vi "getElementText.vi"(8 "error in (no error)":errorcluster, 11 "xwpfTable in":refnum<class "xwpfTable.lvclass">) -> (0 "error out":errorcluster, 2 "Element.Text":string, 3 "xwpfTable out":refnum<class "xwpfTable.lvclass">)   [LabVIEW 2017, in "Word_Specific.lvlib" / "xwpfTable.lvclass"]
uses:
  xwpfTable.lvclass
  Get Cells.Text
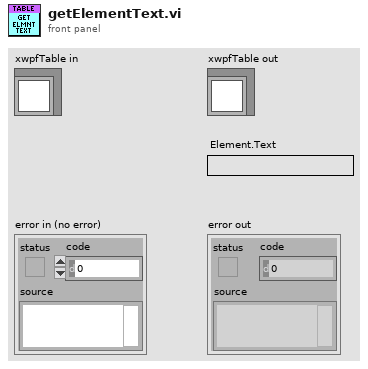
[diagram p1: front panel]
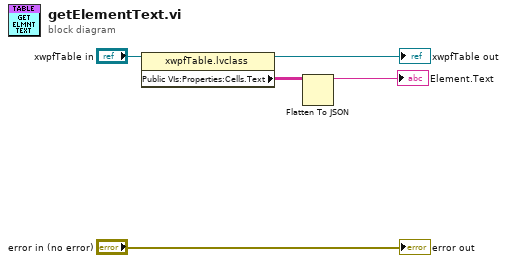
[diagram p0: block diagram]
diagram:
  n1 = property class="xwpfTable.lvclass"(reference="xwpfTable in") -> (reference out=→"xwpfTable out":refnum<class "xwpfTable.lvclass">, "Public VIs:Properties:Cells.Text"=w2:string[][])  [unwired: 1 in, 1 out]
  n2 = Flatten To JSON(anything=w2) -> (JSON string=→"Element.Text":string)  [unwired: 2 in, 1 out]
  "error out" <- "error in (no error)"
